vi "Gyro Rotation.vi"(1 "Current Value":dbl, 2 "Deadband":dbl, 3 "Invert Rotation":bool, 4 "Set Point":dbl) -> (0 "Rotation":dbl)   [LabVIEW 2016]
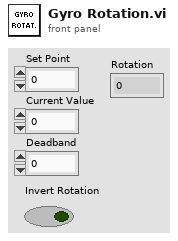
[diagram p1: front panel]
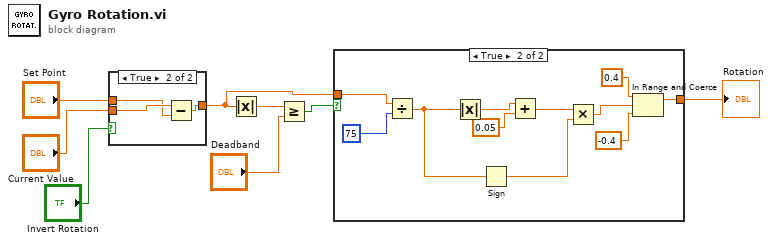
[diagram p0: block diagram]
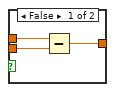
[diagram p2: hidden frame]
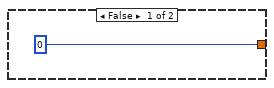
[diagram p3: hidden frame]
diagram:
  n1 = case shown="True" "Invert Rotation" {
    tunnel: [w11 w13] -> w8
    tunnel: "Current Value" -> [w10 w14]
    tunnel: "Set Point" -> [w9 w12]
    frame False {
      n2 = Subtract(x=w9, y=w10) -> (x-y=w11:dbl)
    }
    frame True {
      n3 = Subtract(x=w14, y=w12) -> (x-y=w13:dbl)
    }
  }
  n4 = Absolute Value(x=w8) -> (abs(x)=w6:dbl)
  n5 = Greater Or Equal?(x=w6, y="Deadband") -> (x >= y?=w7:bool)
  n6 = case shown="True" w7 {
    tunnel: [0 w24] -> w5
    tunnel: w8 -> [_ w22]
    frame False {
    }
    frame True {
      n7 = Divide(x=w22, y=75) -> (x/y=w19:dbl)
      n8 = Absolute Value(x=w19) -> (abs(x)=w21:dbl)
      n9 = Sign(1:w19) -> (0:w18:dbl)
      n10 = Add(x=w21, y=0.05) -> (x+y=w17:dbl)
      n11 = Multiply(x=w17, y=w18) -> (x*y=w16:dbl)
      n12 = In Range and Coerce(upper limit=0.4, x=w16, lower limit=-0.4 ("upper limit")) -> (coerced(x)=w24:dbl)  [unwired: 1 out]
    }
  }
  "Rotation" <- w5
